vi "CC Get Data Queue Ref.vi"(8 "error in (no error)":errorcluster) -> (0 "error out":errorcluster, 3 "Data Q":refnum<queue>)   [LabVIEW 2021]
uses:
  SS cluster Data Queue type.ctl
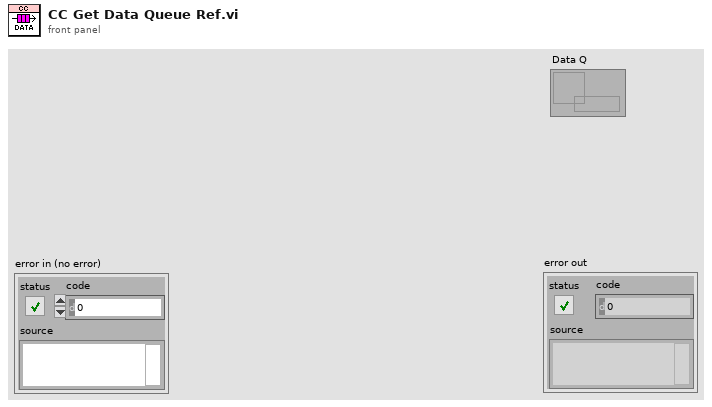
[diagram p1: front panel]
types:
  T1 = typedef "SS cluster Data Queue type.ctl" = cluster{"Source":string, "Type":string, "Data":variant}
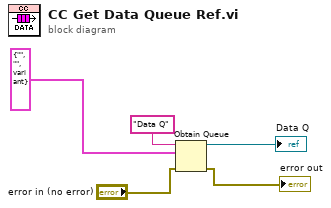
[diagram p0: block diagram]
diagram:
  n1 = Obtain Queue(name (unnamed)="Data Q", element data type=T1 {"Source"="", "Type"="", "Data"=variant} ("Data Q"), error in (no error)="error in (no error)") -> (queue out=→"Data Q":refnum<queue>, error out=→"error out":errorcluster)  [unwired: 2 in, 1 out]
